vi "StoreMainUISettings.vi"(8 "error in (no error)":errorcluster, 11 "MainData in":T1) -> (0 "error out":errorcluster, 3 "MainData out":T1)   [LabVIEW 2019, in "MainController.lvlib"]
uses:
  MainController.lvlib
  Cluster - MainData.ctl
  All Message Queues.ctl
  Cluster - MainControllerMessage.ctl
  Enum - MainState.ctl
  AutoMode/Cluster - AutoModeMessage.ctl
  AutoMode/Enum - AutoModeState.ctl
  ManualMode/Cluster - ManualModeMessageCluster.ctl
  ManualMode/Enum - ManualModeMessage.ctl
  Settings/CTL_MessageCluster.ctl
  Settings/CTL_SettingsMessage.ctl
  EventLogger/Cluster - MessageCluster.ctl
  EventLogger/Enum - Message.ctl
  Cluster - HardwareConfiguration.ctl
  Cluster - LoggingConfiguration.ctl
  Cluster - TestSettings.ctl
  UI State.ctl
  UI Data.ctl
  <vilib>/Utility/config.llb/Write Key (String).vi
  Utilites/Utilities.lvlib
  <vilib>/Utility/config.llb/NI_LVConfig.lvlib
  AutoMode/AutoMode.lvlib
  ManualMode/ManualMode.lvlib
  Settings/Settings.lvlib
  EventLogger/EventLogger.lvlib
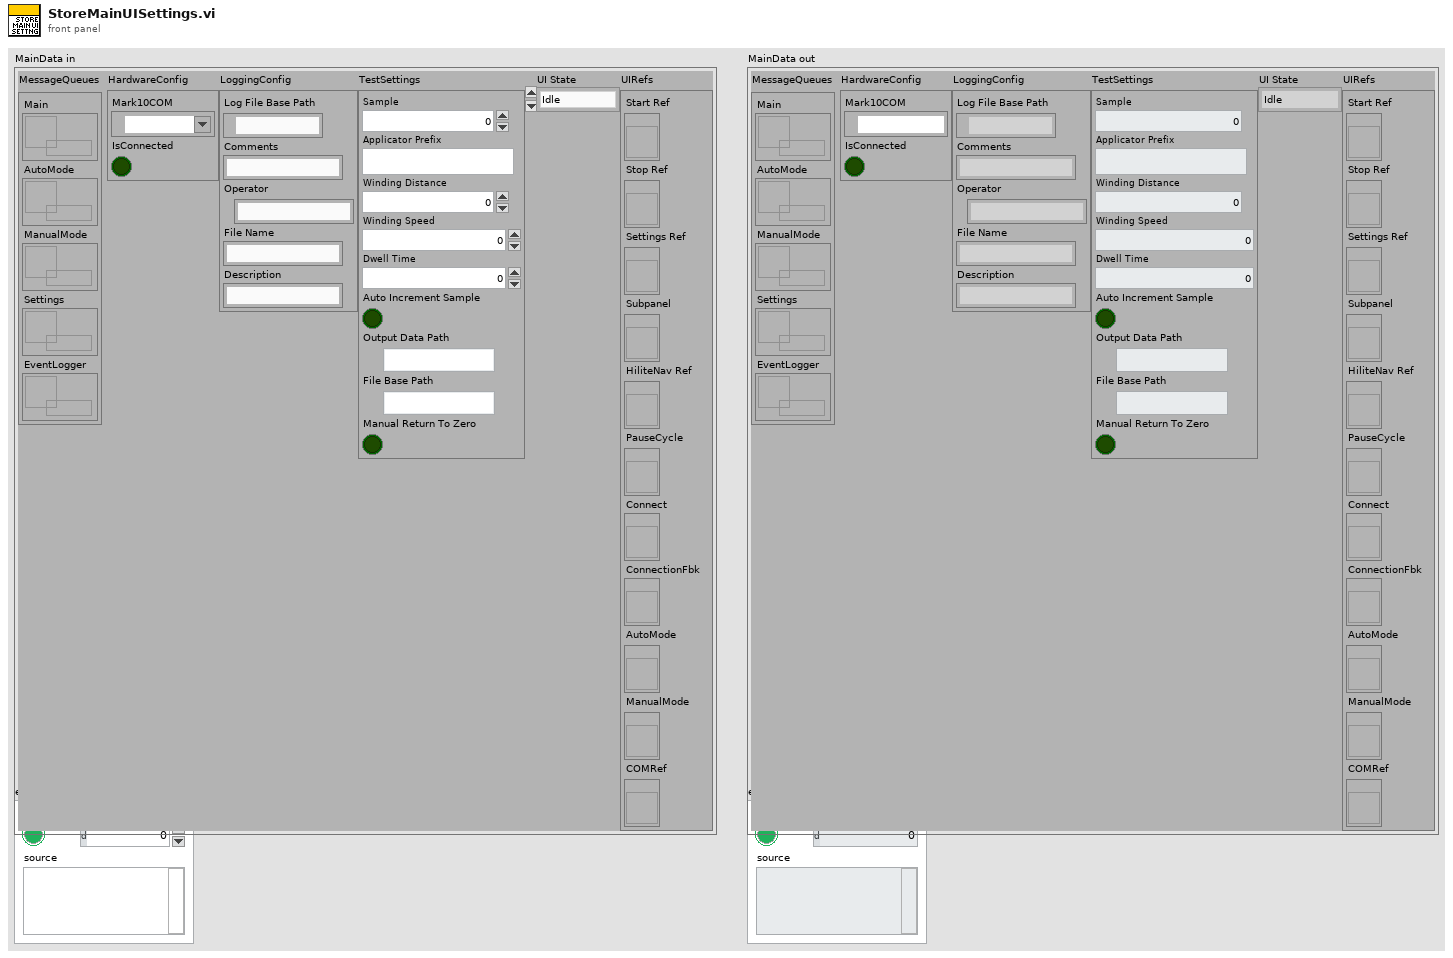
[diagram p1: front panel]
types:
  T1 = typedef "MainController.lvlib/Cluster - MainData.ctl" = cluster{"MessageQueues":T2, "HardwareConfig":T3, "LoggingConfig":T4, "TestSettings":T5, "UI State":T6, "UIRefs":T7}
  T2 = typedef "MainController.lvlib/All Message Queues.ctl" = cluster{"Main":refnum<queue>, "AutoMode":refnum<queue>, "ManualMode":refnum<queue>, "Settings":refnum<queue>, "EventLogger":refnum<queue>}
  T3 = typedef "MainController.lvlib/Cluster - HardwareConfiguration.ctl" = cluster{"Mark10COM":refnum<visa-resource-name>, "IsConnected":bool}
  T4 = typedef "MainController.lvlib/Cluster - LoggingConfiguration.ctl" = cluster{"Log File Base Path":path, "Comments ":string, "Operator":string, "File Name":string, "Description":string}
  T5 = typedef "MainController.lvlib/Cluster - TestSettings.ctl" = cluster{"Sample":u32, "Applicator Prefix":string, "Winding Distance":dbl, "Winding Speed":dbl, "Dwell Time":dbl, "Auto Increment Sample":bool, "Output Data Path":path, "File Base Path":path, "Manual Return To Zero":bool}
  T6 = typedef "MainController.lvlib/UI State.ctl" = enum16{"Idle", "AutoIdle", "AutoRunning", "ManualMode", "Settings"}
  T7 = typedef "MainController.lvlib/UI Data.ctl" = cluster{"Start Ref":refnum<vi>, "Stop Ref":refnum<vi>, "Settings Ref":refnum<vi>, "Subpanel":refnum<vi>, "HiliteNav Ref":refnum<vi>, "PauseCycle":refnum<vi>, "Connect":refnum<vi>, "ConnectionFbk":refnum<vi>, "AutoMode":refnum<vi>, "ManualMode":refnum<vi>, "COMRef":refnum<vi>}
  T8 = typedef "NI_LVConfig.lvlib/Config Data RefNum.ctl" = refnum<k1>
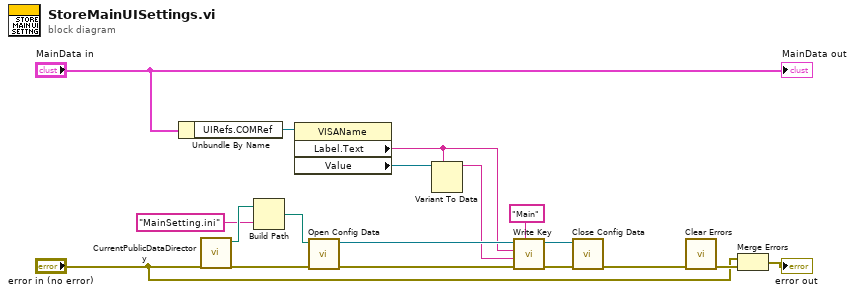
[diagram p0: block diagram]
diagram:
  n1 = Unbundle By Name("MainData in") -> ("UIRefs.COMRef"=w8:refnum<vi>)
  n2 = call "CurrentPublicDataDirectory.vi"() -> ("Public App Directory"=w15:path)  [unwired: 11 in]
  n3 = Build Path(base path=w15, name or relative path="MainSetting.ini") -> (appended path=w13:path)
  n4 = property class="VISAName"(reference=w8) -> ("Label.Text"=w2:string, "Value"=w3:refnum<visa-resource-name>)  [unwired: 1 in, 2 out]
  n5 = call <vilib>:"Open Config Data.vi"("error in (no error)"="error in (no error)", "configuration file path"=w13) -> ("error out"=w16:errorcluster, "refnum"=w11:T8)  [unwired: 7 in, 1 out]
  n6 = Variant To Data(type=w2, Variant=w3) -> (data=w1:string)  [unwired: 1 in, 1 out]
  n7 = call-poly <vilib>:"Write Key.vi"("section"="Main", "error in (no error)"=w16, "value"=w1, "key"=w2, "refnum"=w11) -> ("error out"=w12:errorcluster, "refnum out"=w10:T8)  [unwired: 4 in, 1 out]
  n8 = call <vilib>:"Close Config Data.vi"("error in (no error)"=w12, "refnum"=w10) -> ("error out"=w7:errorcluster)  [unwired: 8 in, 1 out]
  n9 = call <vilib>:"Clear Errors.vi"("error in (no error)"=w7) -> ("error out"=w6:errorcluster)  [unwired: 5 in, 1 out]
  n10 = Merge Errors("error in (no error)", w6) -> (→"error out":errorcluster)
  "MainData out" <- "MainData in"
